vi "Host VI.vi"() -> ()   [LabVIEW 2016]
uses:
  <vilib>/FPGAPlugInAG/sbRIO-9636/niLvFpga_Open_sbRIO-9636.vi
  <vilib>/Utility/error.llb/Error Cluster From Error Code.vi
  <vilib>/rvi/errors/niLvFpgaAdjustHostInterfaceError.vi
  <vilib>/FPGAPlugInAG/sbRIO-9636/niLvFpga_Close_sbRIO-9636.vi
  <vilib>/rvi/interface/nirviOpenFPGA/nirviOpenFPGA.xnode
  FPGA Bitfiles/Practice_FPGATarget_TEST_+EIwWHtjPLs.lvbitx
  TEST.vi
  <vilib>/rvi/interface/nirviReadWriteControl/nirviReadWriteControl.xnode
  <vilib>/rvi/interface/nirviCloseFPGA/nirviCloseFPGA.xnode
  NiFpgaLv.dll
panel:
  out "Filtered Sine":i16(graph)
  out "Measured Sine":i16(graph)
  in  "stop":bool
  out "Clean Sine":i16(graph)
  out "Noisy Sine":i16(graph)
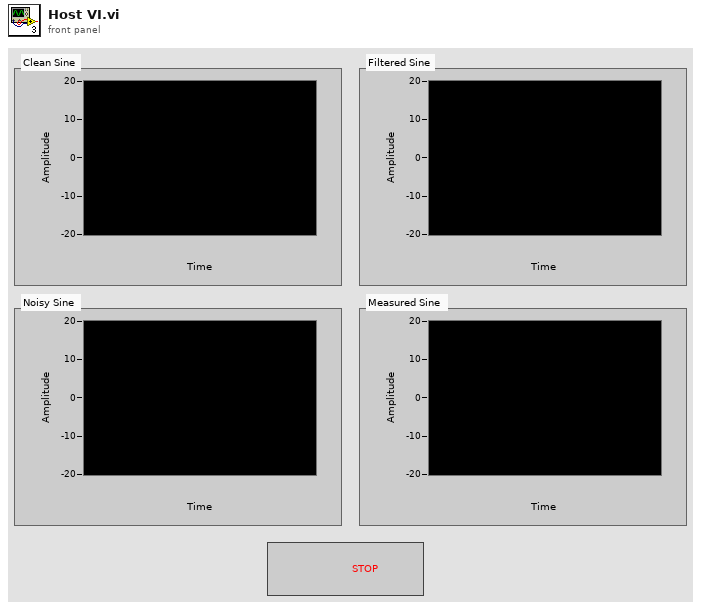
[diagram p1: front panel]
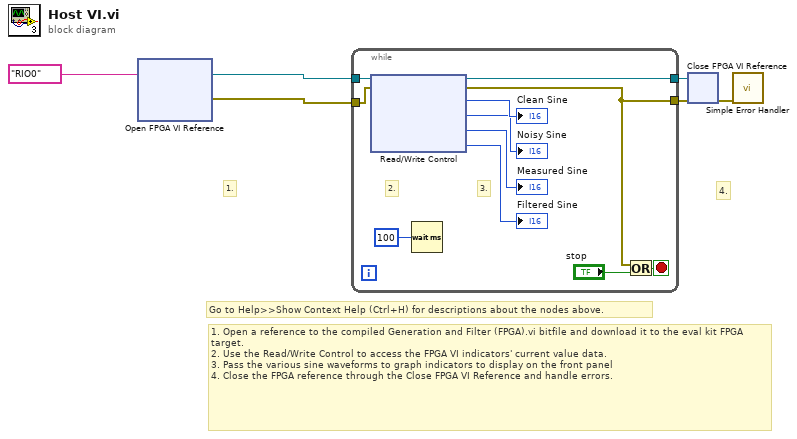
[diagram p0: block diagram]
diagram:
  # "4."
  # "1."
  # "Go to Help>>Show Context Help (Ctrl+H) for descriptions about the nodes above."
  # "1. Open a reference to the compiled Generation and Filter (FPGA).vi bitfile and download it to the eval kit FPGA target.\n2. Use the Read/Write Control to access the FPGA VI indicators' current value data.\n3. Pass the various sine waveforms to graph indicators to display on the front panel\n4. Close the FPGA reference through the Close FPGA VI Reference and handle errors."
  n1 = xnode "Open FPGA VI Reference"("resource name"=tag "RIO0") -> ("FPGA VI Reference Out"=w6:refnum<k20>, "error out"=w4:errorcluster)  [unwired: 1 in]
  n2 = while "Host" {
    tunnel: w6 -> [w17]
    tunnel: w4 -> [w10]
    tunnel: [w9] -> w3
    tunnel: [w7] -> w2
    stop <- w12 stop-if-true
    # "3."
    # "2."
    n3 = xnode "Read/Write Control"("FPGA VI Reference In"=w17, "error in"=w10) -> ("FPGA VI Reference Out"=w9:refnum<k20>, "error out"=w7:errorcluster, "Clean Sine"=→"Clean Sine":i16, "Noisy Sine"=→"Noisy Sine":i16, "Measured Sine"=→"Measured Sine":i16, "Filtered Sine"=→"Filtered Sine":i16)
    n4 = Wait (ms)(milliseconds to wait=u32 100) -> ()  [unwired: 1 out]
    n5 = Or(x=w7, y="stop") -> (x .or. y?=w12:bool)
  }
  n6 = xnode "Close FPGA VI Reference"("FPGA VI Reference In"=w3, "error in"=w2) -> ("error out"=w5:errorcluster)
  n7 = call <vilib>:"Simple Error Handler.vi"("error in (no error)"=w5) -> ()  [unwired: 1 in, 8 out]
